vi "CSMLS - Remove Loop Tag to Break.vi"(11 "States Queue":string) -> (3 "Remaining States":string)   [LabVIEW 2017, in "CSM Loop Support.lvlib"]
doc: "Stops the loop by removing the `<loop>` tag.\n\n<b>Example</b>:\n\nIf the following messages exist in the CSM message queue, executing the current API operation will remove the messages where the comments are located.\n\n```\nDAQ: Acquire\nDAQ: Continuous Check -><loop> // Will be removed\nDAQ: Stop\nDAQ: Close\n```\n\nThis is equivalent to still executing the current DAQ operation, and then entering stop and release.\n\n-- <b>Controls</b> --\n- <b>States Queue</b>: Connect the entire state queue to this input.\n\n-- <b>Indicators</b> --\n- <b>Remaining States</b>: The remaining message queue."
uses:
  CSM Loop Support.lvlib
  Communicable State Machine.lvlib
  _Shared/CSM Shared.lvlib
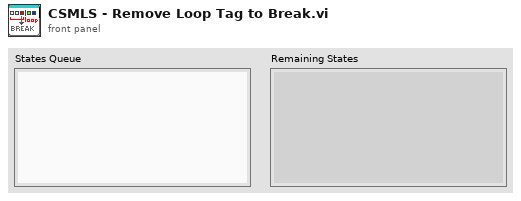
[diagram p1: front panel]
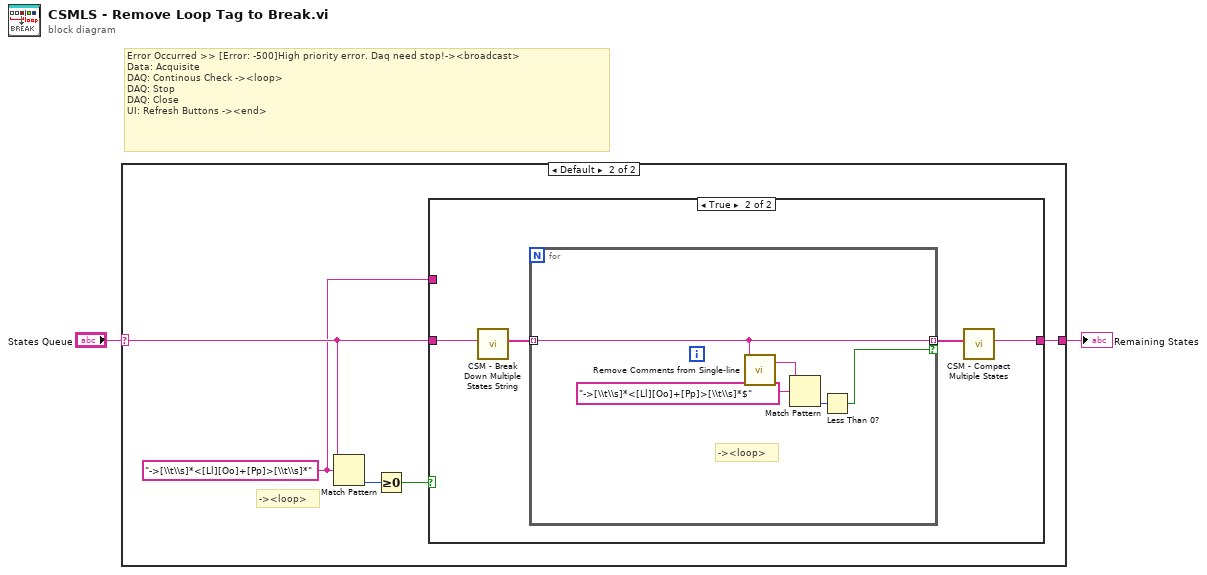
[diagram p0: block diagram]
diagram:
  # "Error Occurred >> [Error: -500]High priority error. Daq need stop!-><broadcast>\nData: Acquisite\nDAQ: Continous Check -><loop>\nDAQ: Stop\nDAQ: Close\nUI: Refresh Buttons -><end>"
  n1 = case shown="Default" "States Queue" {
    selector: "States Queue" -> [w3 w6]
    tunnel: [w3 w8] -> w2
    frame "" {
    }
    frame Default {
      w4 = "->[\\t\\s]*<[Ll][Oo]+[Pp]>[\\t\\s]*" ("regular expression")
      # "-><loop>"
      n2 = Match Pattern(string=w6, regular expression=w4) -> (offset past match=w7:i32)  [unwired: 1 in, 3 out]
      n3 = Greater Or Equal To 0?(x=w7) -> (x >= 0?=w5:bool)
      n4 = case shown="True" w5 {
        tunnel: [w9 w13] -> w8
        tunnel: w6 -> [w9 w12]
        tunnel: w4 -> [_ _]
        frame False {
        }
        frame True {
          n5 = call "CSM - Break Down Multiple States String.vi"("States"=w12) -> ("Multiple States"=w11:string[])  [unwired: 10 in]
          n6 = for {
            tunnel: [w15] -> w10 mode=indexing if=w16
            tunnel: w11 -> [w15] mode=indexing
            # "-><loop>"
            n7 = call "Remove Comments from Single-line.vi"("single-line text"=w15) -> ("single-line text without comments"=w14:string)  [unwired: 2 in]
            n8 = Match Pattern(string=w14, regular expression="->[\\t\\s]*<[Ll][Oo]+[Pp]>[\\t\\s]*$") -> (offset past match=w17:i32)  [unwired: 1 in, 3 out]
            n9 = Less Than 0?(x=w17) -> (x < 0?=w16:bool)
          }
          n10 = call "CSM - Compact Multiple States.vi"("Multiple States"=w10) -> ("States"=w13:string)  [unwired: 9 in]
        }
      }
    }
  }
  "Remaining States" <- w2
